vi "扫码状态查询.vi"(8 "error in":errorcluster, 9 "运行状态":string, 10 "sn":refnum<vi>, 11 "MB_实体":refnum<class "Modbus Master.lvclass">) -> (0 "输出簇":errorcluster)   [LabVIEW 2020]
uses:
  <vilib>/NI/Modbus Library/API/Master/Modbus Master.lvclass
  Global.vi
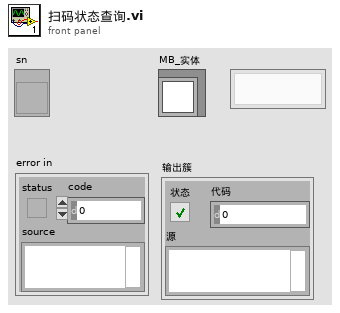
[diagram p1: front panel]
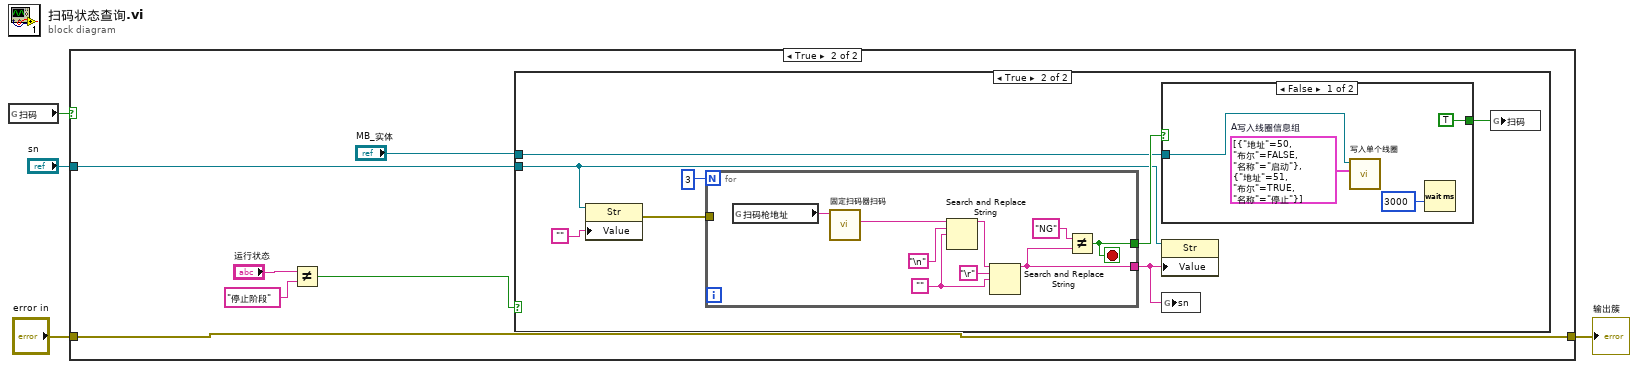
[diagram p0: block diagram]
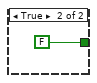
[diagram p4: hidden frame]
diagram:
  n1 = global read "Global.vi" "扫码"() -> (w4:bool)
  n2 = case shown="True" w4 {
    tunnel: "sn" -> [_ w9]
    tunnel: "error in" -> [_ w8]
    tunnel: [_ w8] -> w1
    frame False {
    }
    frame True {
      n3 = Not Equal?(x="运行状态", y="停止阶段" ("名称")) -> (x != y?=w5:bool)
      n4 = case shown="True" w5 {
        tunnel: "MB_实体" -> [_ w15]
        tunnel: w9 -> [_ w13]
        frame False {
        }
        frame True {
          n5 = property class="Str"(reference=w13, "Value"="") -> (error out=w11:errorcluster)  [unwired: 1 in, 1 out]
          n6 = for {
            N: 3 -> [_]
            tunnel: [w25] -> w17
            tunnel: [w24] -> w16
            tunnel: w11 -> [_]
            stop <- w24 stop-if-true
            w27 = ""
            n7 = global read "Global.vi" "扫码枪地址"() -> (w32:string)
            n8 = call "固定扫码器扫码.vi"("VISA资源名称"=w32) -> ("响应"=w31:string)  [unwired: 9 in, 1 out]
            n9 = Search and Replace String(input string=w31, search string="\n", replace string=w27) -> (result string=w30:string)  [unwired: 5 in, 3 out]
            n10 = Search and Replace String(input string=w30, search string="\r", replace string=w27) -> (result string=w25:string)  [unwired: 5 in, 3 out]
            n11 = Not Equal?(x="NG", y=w25) -> (x != y?=w24:bool)
          }
          n12 = case shown="False" w16 {
            tunnel: w15 -> [w22 _]
            tunnel: [TRUE ("扫码") FALSE ("扫码")] -> w14
            frame False {
              w20 = cluster{"地址":u16, "布尔":bool, "名称":string}[] [{"地址"=50, "布尔"=FALSE, "名称"="启动"}, {"地址"=51, "布尔"=TRUE, "名称"="停止"}]  # A写入线圈信息组
              n13 = call "写入单个线圈.vi"("写入线圈信息组"=w20, "MB_实体"=w22) -> ()  [unwired: 8 in, 2 out]
              n14 = Wait (ms)(milliseconds to wait=u32 3000) -> ()  [unwired: 1 out]
            }
            frame True {
            }
          }
          n15 = property class="Str"(reference=w13, "Value"=w17) -> ()  [unwired: 1 in, 2 out]
          n16 = global write "Global.vi" "sn"(w17) -> ()
          n17 = global write "Global.vi" "扫码"(w14) -> ()
        }
      }
    }
  }
  "输出簇" <- w1
